vi "Robot Global Data.vi"() -> ()   [LabVIEW 2014]
doc: "This global VI can contain as many global variables as you need. Place a control on the panel, give it a good name. To read or write to it from a VI, drag the icon to the diagram of that VI. You can also drag from the project. Click on the node to change which global you access. You shouldn't have multiple locations writing to a global or it will cause a race-condition."
uses:
  <vilib>/Rock Robotics/WPI/Camera/WPI_CameraImageSize.ctl
  <vilib>/Rock Robotics/WPI/DriverStation/WPI_DriverStationRobotMode2.ctl
panel:
  in  "Lift PID Enabled?":bool
  out "Elevator Number of rotations":dbl
  out "Elevator Previous Rotation":dbl
  out "Power Distribution Board Slot for Elevator Motor":u8
  out "Number of items carrying (Totes & RCs)":dbl
  in  "Elevator Clear Tote State":T1(ring)
  in  "Elevator Carry RC State":T2(ring)
  in  "Elevator State Setting":T3(ring)
  in  "Elevator Bottom State":T4(ring)
  in  "Claw Close State":T5(ring)
  in  "Claw Open State":T6(ring)
  in  "Claw State Setting":T7(ring)
  in  "Was Claw OPEN Button Pressed Last Time":bool
  in  "Was Claw CLOSE Button Pressed Last Time":bool
  out "Autonomous Selected":dbl
  in  "Lift Computer Controlled":bool
  out "Lift Set Point":dbl
  in  "Robot Mode":T8=enum."Finish"
  in  "image size":T9=enum."320x240"
  in  "Enable Vision":bool=TRUE
  # "Lift Related"
  # "Claw Related"
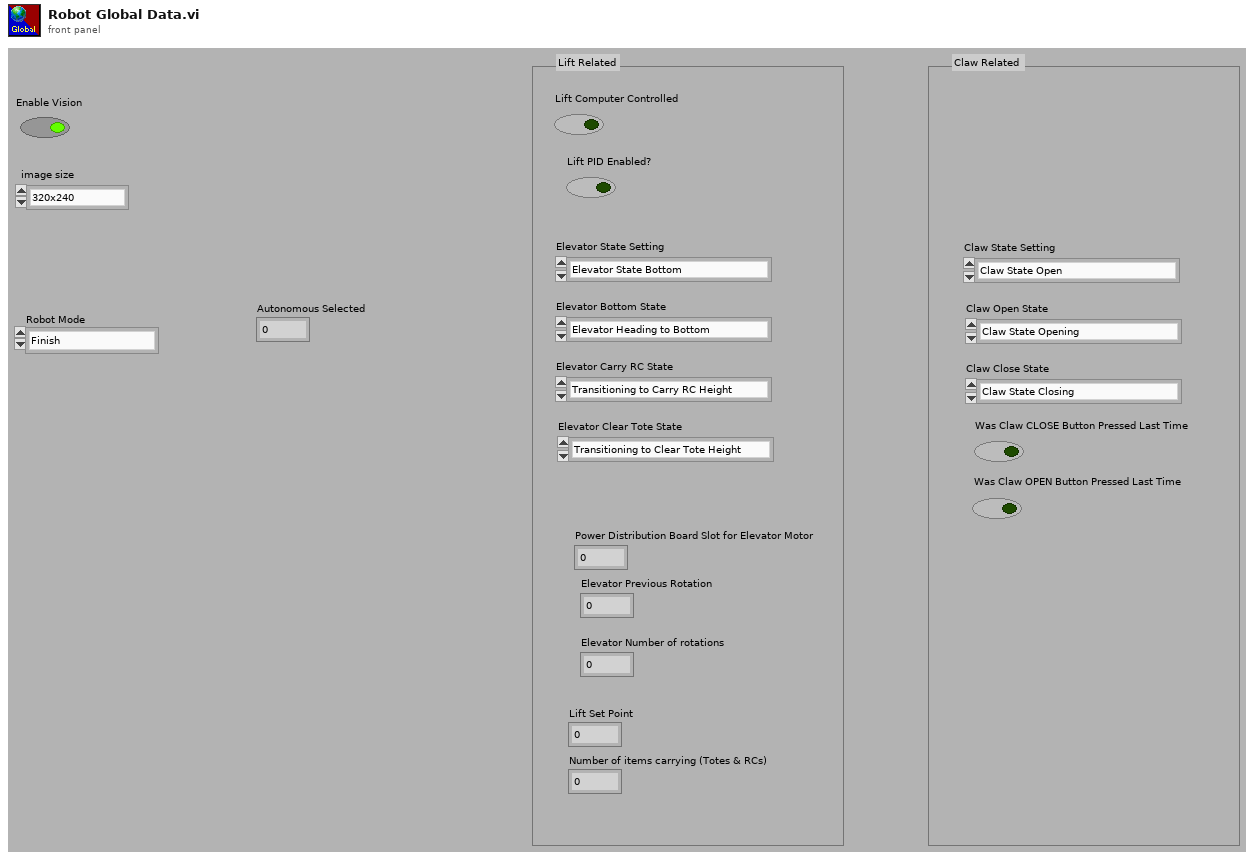
[diagram p1: front panel]
types:
  T1 = enum16{"Transitioning to Clear Tote Height", "At Clear Tote Height"}
  T2 = enum16{"Transitioning to Carry RC Height", "At Carry RC Height"}
  T3 = enum16{"Elevator State Bottom", "Elevator State Clear a Tote", "Elevator State Carry a  RC", "Elevator do Nothing"}
  T4 = enum16{"Elevator Heading to Bottom", "Elevator Reached Bottom"}
  T5 = enum16{"Claw State Closing", "Claw State Closed", "Squeeze"}
  T6 = enum16{"Claw State Opening", "Claw State Opened"}
  T7 = enum16{"Claw State Open", "Claw State Closed", "Claw State Do Nothing", "Squeeze Hard"}
  T8 = typedef "WPI_DriverStationRobotMode2.ctl" = enum16{"Autonomous Disabled", "Autonomous Enabled", "Teleop Disabled", "Teleop Enabled", "Disconnected", "Finish", "Test Disabled", "Test Enabled", "Emergency Stopped"}
  T9 = typedef "WPI_CameraImageSize.ctl" = enum16{"640x480", "320x240", "160x120", "Custom"}
diagram:
